vi "Write Digital Outptus.vi"(0 "Acquisition Trigger Output Terminal 2":T1, 1 "Shutter Output Terminal":T1, 2 "Shutter Output Value":bool, 4 "Acquisition Trigger Output Terminal":T1, 6 "Beam Clock Output Terminal 2":T1, 7 "Digital Outputs":T2, 8 "Beam Clock Output Terminal":T1, 9 "Frame Clock Ouput Terminal 2":T1, 10 "Frame Clock Ouput Terminal":T1, 11 "Period Clock Ouput Terminal":T1) -> ()   [LabVIEW 2014]
uses:
  Trigger Output Terminals.ctl
  Trigger Output Signals.ctl
  <vilib>/rvi/eio/common/nirviEmuTemplateMethod_errors.vi
  <vilib>/eio/EIONode/EIONode.xnode
  <vilib>/eio/EIOMethodNode/EIOMethodNode.xnode
panel:
  # "Copyright 2014 Vidrio Technologies\nScanImage 5 software is licensed under the Apache License, Version 2.0 (the \"License\"); you may not use any files contained\nwithin the ScanImage 5 release except in compliance with the License. You may obtain a copy of the License at\n http://www.apache.org/licenses/LICENSE-2.0\nUnless required by applicable law or agreed to in writing, software distributed under the License is distributed on an\n\"AS IS\" BASIS, WITHOUT WARRANTIES OR CONDITIONS OF ANY KIND, either express or implied. See the License for the\n specific language governing permissions and limitations under the License."
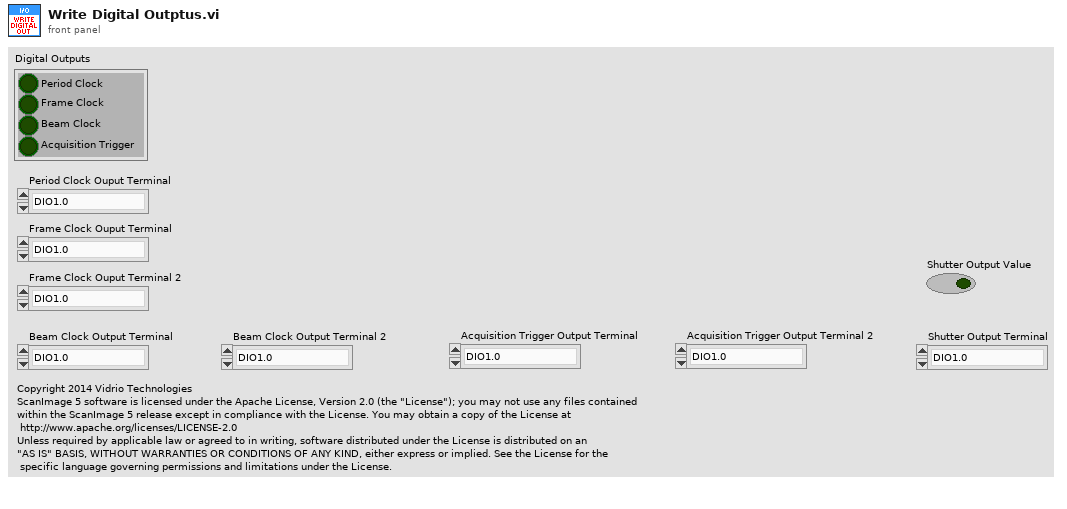
[diagram p1: front panel]
types:
  T1 = typedef "Trigger Output Terminals.ctl" = enum8{"DIO1.0", "DIO1.1", "DIO1.2", "DIO1.3", "PXI_Trig0", "PXI_Trig1", "PXI_Trig2", "PXI_Trig3", "PXI_Trig4", "PXI_Trig5", "PXI_Trig6", "PXI_Trig7", ""}
  T2 = typedef "Trigger Output Signals.ctl" = cluster{"Period Clock":bool, "Frame Clock":bool, "Beam Clock":bool, "Acquisition Trigger":bool}
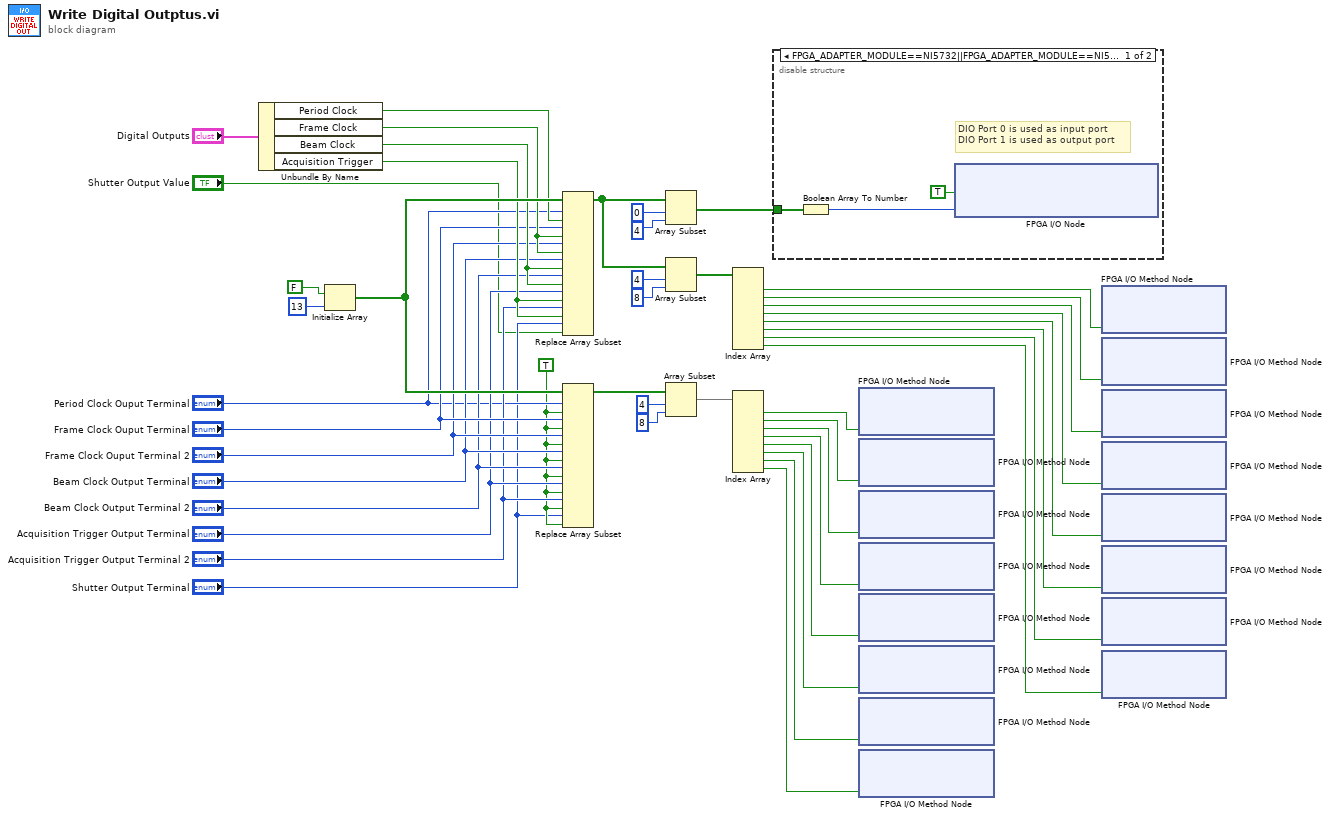
[diagram p0: block diagram]
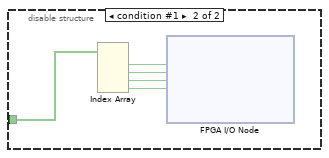
[diagram p2: hidden frame]
diagram:
  w4 = TRUE ("new element/subarray")
  n1 = Unbundle By Name("Digital Outputs") -> ("Period Clock"=w6:bool, "Frame Clock"=w15:bool, "Beam Clock"=w14:bool, "Acquisition Trigger"=w13:bool)
  n2 = Initialize Array(FALSE, 13 ("dimension size")) -> (w29:bool[])
  n3 = Replace Array Subset(array=w29, new element #1=w6, index #1="Period Clock Ouput Terminal", new element #2=w15, index #2="Frame Clock Ouput Terminal", new element #3=w15, index #3="Frame Clock Ouput Terminal 2", new element #4=w14, index #4="Beam Clock Output Terminal", new element #5=w14, index #5="Beam Clock Output Terminal 2", new element #6=w13, index #6="Acquisition Trigger Output Terminal", new element #7=w13, index #7="Acquisition Trigger Output Terminal 2", new element #8="Shutter Output Value", index #8="Shutter Output Terminal") -> (w26:bool[])
  n4 = Replace Array Subset(array=w29, new element #1=w4, index #1="Period Clock Ouput Terminal", new element #2=w4, index #2="Frame Clock Ouput Terminal", new element #3=w4, index #3="Frame Clock Ouput Terminal 2", new element #4=w4, index #4="Beam Clock Output Terminal", new element #5=w4, index #5="Beam Clock Output Terminal 2", new element #6=w4, index #6="Acquisition Trigger Output Terminal", new element #7=w4, index #7="Acquisition Trigger Output Terminal 2", new element #8=w4, index #8="Shutter Output Terminal") -> (w41:bool[])
  n5 = Array Subset(array=w26, index=0, length=4) -> (w1:bool[])
  n6 = Array Subset(array=w26, index=4, length=8) -> (w25:bool[])
  n7 = Array Subset(array=w41, index=4, length=8) -> (w38:bool[])
  n8 = Index Array(array=w25) -> (element #1=w24:bool, element #2=w23:bool, element #3=w22:bool, element #4=w21:bool, element #5=w20:bool, element #6=w19:bool, element #7=w18:bool, element #8=w17:bool)  [unwired: 8 in]
  n9 = Index Array(array=w38) -> (element #1=w37:bool, element #2=w36:bool, element #3=w35:bool, element #4=w34:bool, element #5=w33:bool, element #6=w32:bool, element #7=w31:bool, element #8=w30:bool)  [unwired: 8 in]
  n10 = disable-structure shown="FPGA_ADAPTER_MODULE==NI5732||FPGA_ADAPTER_MODULE==NI5734, Default" {
    disable-tunnel: w1 -> [w47 w53]
    frame condition #0 (active) {
      # "DIO Port 0 is used as input port\nDIO Port 1 is used as output port"
      n11 = Boolean Array To Number(Boolean array=w47) -> (number=w46:u8)
      n12 = xnode "FPGA I/O Node"("IO Module\\DIO Port 1 WE"=TRUE ("IO Module\\DIO Port 1 WE"), "IO Module\\DIO Port 1 Wr Data"=w46) -> ()  [unwired: 2 in, 2 out]
    }
    frame condition #1 {
      n13 = Index Array(array=w53) -> (element #1=w52:bool, element #2=w51:bool, element #3=w50:bool, element #4=w49:bool)  [unwired: 4 in]
      n14 = xnode "FPGA I/O Node"("IO Module\\D0 0"=w52, "IO Module\\D0 1"=w51, "IO Module\\D0 2"=w50, "IO Module\\D0 3"=w49) -> ()  [unwired: 4 in, 4 out]
    }
  }
  n15 = xnode "FPGA I/O Method Node"("Enable"=w37) -> ()  [unwired: 1 in, 1 out]
  n16 = xnode "FPGA I/O Method Node"("Enable"=w36) -> ()  [unwired: 1 in, 1 out]
  n17 = xnode "FPGA I/O Method Node"("Enable"=w35) -> ()  [unwired: 1 in, 1 out]
  n18 = xnode "FPGA I/O Method Node"("Enable"=w34) -> ()  [unwired: 1 in, 1 out]
  n19 = xnode "FPGA I/O Method Node"("Enable"=w33) -> ()  [unwired: 1 in, 1 out]
  n20 = xnode "FPGA I/O Method Node"("Enable"=w32) -> ()  [unwired: 1 in, 1 out]
  n21 = xnode "FPGA I/O Method Node"("Enable"=w31) -> ()  [unwired: 1 in, 1 out]
  n22 = xnode "FPGA I/O Method Node"("Enable"=w30) -> ()  [unwired: 1 in, 1 out]
  n23 = xnode "FPGA I/O Method Node"("Data"=w24) -> ()  [unwired: 1 in, 1 out]
  n24 = xnode "FPGA I/O Method Node"("Data"=w23) -> ()  [unwired: 1 in, 1 out]
  n25 = xnode "FPGA I/O Method Node"("Data"=w22) -> ()  [unwired: 1 in, 1 out]
  n26 = xnode "FPGA I/O Method Node"("Data"=w21) -> ()  [unwired: 1 in, 1 out]
  n27 = xnode "FPGA I/O Method Node"("Data"=w20) -> ()  [unwired: 1 in, 1 out]
  n28 = xnode "FPGA I/O Method Node"("Data"=w19) -> ()  [unwired: 1 in, 1 out]
  n29 = xnode "FPGA I/O Method Node"("Data"=w18) -> ()  [unwired: 1 in, 1 out]
  n30 = xnode "FPGA I/O Method Node"("Data"=w17) -> ()  [unwired: 1 in, 1 out]
